vi "ShooterTEST.vi"(5 "WinchCaseIn":dbl, 8 "OutGearPos":dbl=2.1, 9 "InGearPos":dbl=1.5, 10 "Pot":dbl, 11 "Fire":bool) -> (0 "There?":bool, 1 "WinchCase":i32, 3 "Power":dbl)   [LabVIEW 2013]
panel:
  out "Index":i32
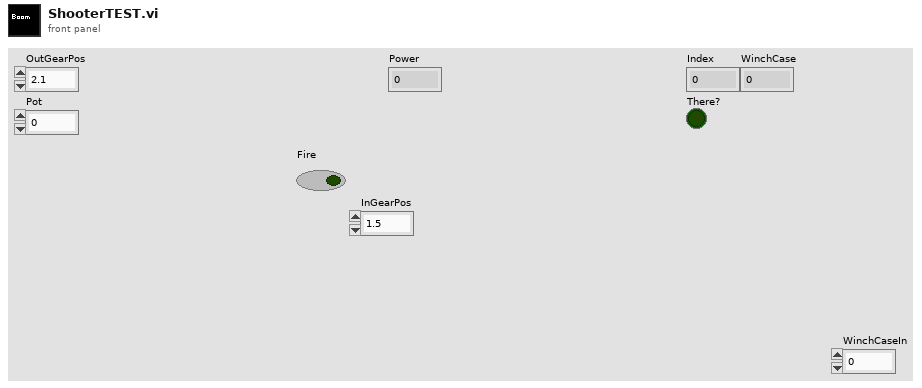
[diagram p1: front panel]
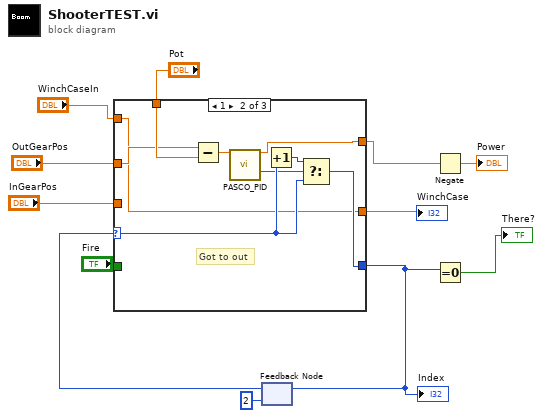
[diagram p0: block diagram]
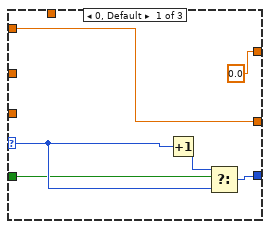
[diagram p2: hidden frame]
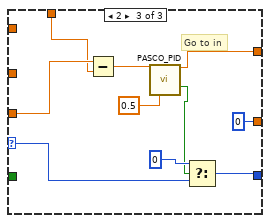
[diagram p3: hidden frame]
diagram:
  n1 = feedback #1(2 ("Numeric")) -> (w10:i32)
  n2 = case shown="1" w10 {
    selector: w10 -> [w16 w25 w35]
    tunnel: [0.0 ("Output") w24 w34] -> w1
    tunnel: "Fire" -> [w15 _ _]
    tunnel: [w18 w27 w37] -> w7
    tunnel: "OutGearPos" -> [_ w20 _]
    tunnel: "InGearPos" -> [_ _ w32]
    tunnel: "Pot" -> [_ w21 w31]
    tunnel: [w13 w19 0 ("WinchCase")] -> w4
    tunnel: "WinchCaseIn" -> [w13 w19 _]
    frame 0, Default {
      n3 = Increment(x=w16) -> (x+1=w17:i32)
      n4 = Select(t=w17, s=w15, f=w16) -> (s? t:f=w18:i32)
    }
    frame 1 {
      # "Got to out"
      n5 = Subtract(x=w20, y=w21) -> (x-y=w22:dbl)
      n6 = call "PASCO_PID.vi"("Delta"=w22) -> ("Output"=w24:dbl, "IsThere"=w23:bool)  [unwired: 13 in]
      n7 = Increment(x=w25) -> (x+1=w26:i32)
      n8 = Select(t=w26, s=w23, f=w25) -> (s? t:f=w27:i32)
    }
    frame 2 {
      # "Go to in"
      n9 = Subtract(x=w32, y=w31) -> (x-y=w30:dbl)
      n10 = call "PASCO_PID.vi"("Delta"=w30, "P Gain"=0.5) -> ("Output"=w34:dbl, "IsThere"=w33:bool)  [unwired: 12 in]
      n11 = Select(t=0, s=w33, f=w35) -> (s? t:f=w37:i32)
    }
  }
  "Index" <- w7
  "WinchCase" <- w4
  n12 = feedback-in #1(w7) -> ()
  n13 = Negate(x=w1) -> (-x=→"Power":dbl)
  n14 = Equal To 0?(x=w7) -> (x = 0?=→"There?":bool)
